vi "Write ID-attribute.vi"(8 "error in (no error)":errorcluster, 10 "ID-attribute":T1, 11 "ID in":refnum<class "ID.lvclass">) -> (0 "error out":errorcluster, 3 "ID out":refnum<class "ID.lvclass">)   [LabVIEW 2013, in "MaterialCharacterization.lvlib" / "ID.lvclass"]
uses:
  ID.lvclass
  Attribute-ID.ctl
  ID.lvclass/ID.ctl
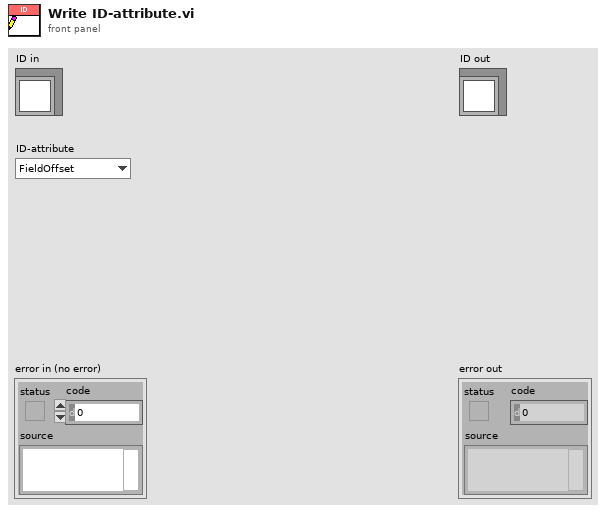
[diagram p1: front panel]
types:
  T1 = typedef "MaterialCharacterization.lvlib/ID.lvclass/Attribute-ID.ctl" = enum16{"FieldOffset", "TransformEnable", "Transform", "Units", "XYCalFactor", "EnableLaser", "JumpDelay", "MarkDelay", "PolyDelay", "LaserOnDelay", "LaserOffDelay", "JumpSpeed", "MarkSpeed", "LaserPowerDelay", "LaserEnableDelay", "LaserPower", "Offset"}
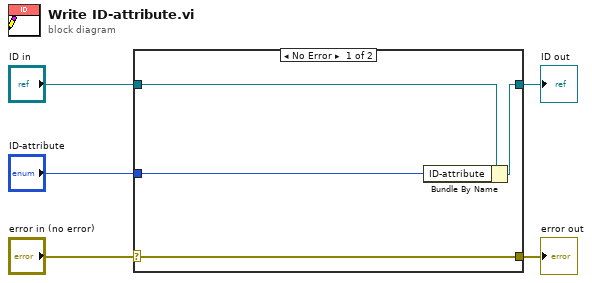
[diagram p0: block diagram]
diagram:
  n1 = case shown="No Error" "error in (no error)" {
    selector: "error in (no error)" -> [w9 w10]
    tunnel: [w9 w10] -> w4
    tunnel: [w7 w11] -> w2
    tunnel: "ID in" -> [w8 w11]
    tunnel: "ID-attribute" -> [w6 _]
    frame No Error {
      n2 = Bundle By Name(cluster=w8, "ID-attribute"=w6) -> (w7:refnum<class "ID.lvclass">)
    }
    frame Error {
    }
  }
  "error out" <- w4
  "ID out" <- w2
